vi "Insert.vi"(8 "error in (no error)":errorcluster caption="错误输入（无错误）", 11 "SQL Department 输入":refnum<class "SQL Department.lvclass">) -> (0 "error out":errorcluster caption="错误输出", 2 "字符串":string, 3 "SQL Department 输出":refnum<class "SQL Department.lvclass">)   [LabVIEW 2017, in "SQL Department.lvclass"]
uses:
  SQL Department.lvclass
  Abstract Department/Abstract Department.lvclass
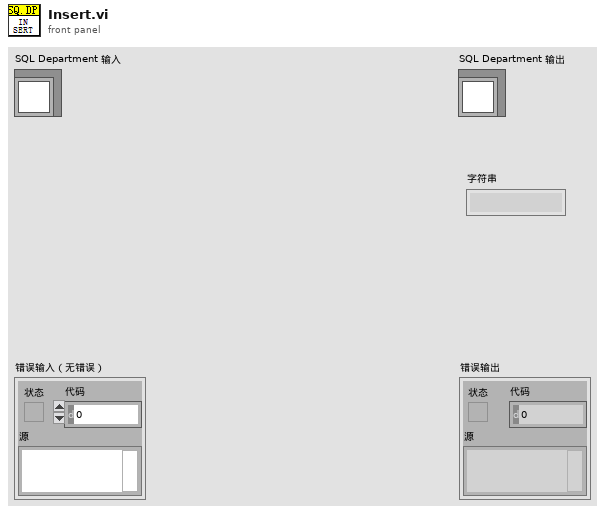
[diagram p1: front panel]
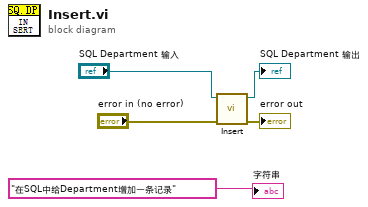
[diagram p0: block diagram]
diagram:
  n1 = call-parent "Insert.vi"("error in (no error)"="error in (no error)", "Abstract Department 输入"="SQL Department 输入") -> ("error out"=→"error out":errorcluster, "Abstract Department 输出"=→"SQL Department 输出":refnum<class "SQL Department.lvclass">)  [unwired: 7 in, 1 out]
  "字符串" <- "在SQL中给Department增加一条记录" ("字符串")
